vi "R_rdp.vi"(1 "install path":path=path "C:/Program Files (x86)/National Instruments/LabLinda", 5 "IN VARIANT":variant, 7 "Ip":string, 9 "Name in":string, 11 "error in (no error)":errorcluster) -> (6 "OUT VARIANT":variant, 10 "Operation Ok":bool, 15 "error out":errorcluster)   [LabVIEW 2015]
doc: "REMOTE rdp."
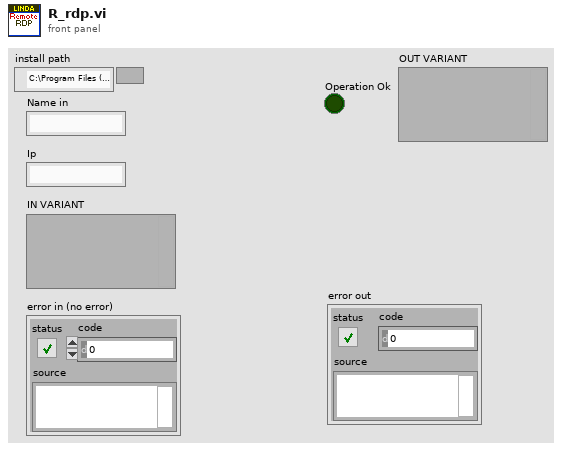
[diagram p1: front panel]
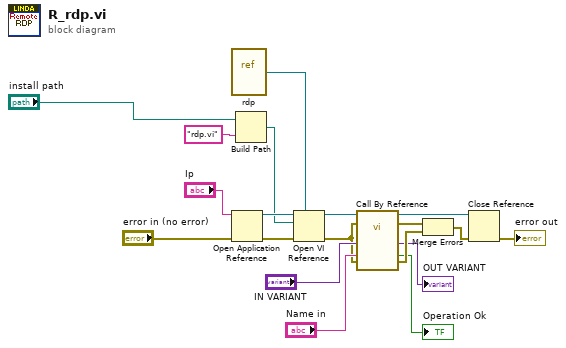
[diagram p0: block diagram]
diagram:
  n1 = vi-ref "rdp.vi"() -> (w1:refnum<vi>)
  n2 = Open Application Reference(8:"error in (no error)", 11:"Ip") -> (0:w14:errorcluster, 3:w17:refnum<vi>)  [unwired: 2 in]
  n3 = Build Path(base path="install path", name or relative path="rdp.vi") -> (appended path=w15:path)
  n4 = Open VI Reference(type specifier VI Refnum (for type only)=w1, application reference (local)=w17, vi path=w15, error in (no error)=w14) -> (vi reference=w2:refnum<vi>, error out=w7:errorcluster)  [unwired: 2 in]
  n5 = call-by-ref "?"(reference=w2, error in=w7, "IN VARIANT"="IN VARIANT", "Name in"="Name in", 11:"error in (no error)"=w7) -> (reference out=w10:refnum<vi>, error out=w13:errorcluster, "OUT VARIANT"=→"OUT VARIANT":variant, "Valid data"=→"Operation Ok":bool, 15:"error out"=w12:errorcluster)  [unwired: 10 in]
  n6 = Merge Errors(w13, w12) -> (w11:errorcluster)
  n7 = Close Reference(reference=w10, error in (no error)=w11) -> (error out=→"error out":errorcluster)
